vi "FTW-TestExecutive-Core_StepType_ConfigVI.vi"(0 "Step Actor":refnum<vi>, 1 "Other Config Items":string="{}", 5 "Inbox Address":string="inproc://*") -> (4 "Base Config String":string="{}")   [LabVIEW 2015, in "FTW-TestExecutive-Core.lvclass"]
uses:
  FTW-TestExecutive-Core.lvclass
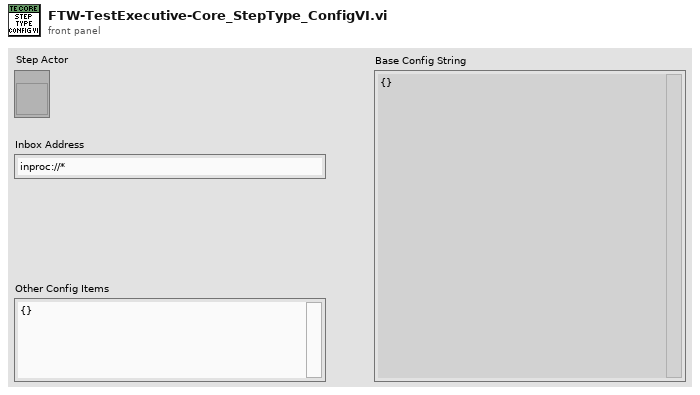
[diagram p1: front panel]
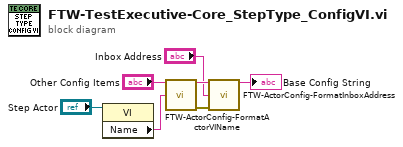
[diagram p0: block diagram]
diagram:
  n1 = property class="VI"(reference="Step Actor") -> ("Name"=w1:string)  [unwired: 1 in, 2 out]
  n2 = call "FTW-ActorConfig-FormatActorVIName.vi"("FTW Config String In"="Other Config Items", "Actor VI Name"=w1) -> ("FTW Config String"=w5:string, "error out"=w4:errorcluster)  [unwired: 12 in]
  n3 = call "FTW-ActorConfig-FormatInboxAddress.vi"("FTW Config String In"=w5, "Inbox Address"="Inbox Address", "error in"=w4) -> ("FTW Config String"=→"Base Config String":string)  [unwired: 11 in, 1 out]
